vi "Tusk.ValidateName.vi"(8 "error in (no error)":errorcluster, 10 "Name":string, 11 "Tusk in":refnum<class "Tusk.lvclass">) -> (0 "error out":errorcluster, 3 "Tusk out":refnum<class "Tusk.lvclass">)   [LabVIEW 2018, in "Application.lvlib" / "Tusk.lvclass"]
uses:
  Tusk.lvclass
  Exceptions Class/Exceptions.lvclass
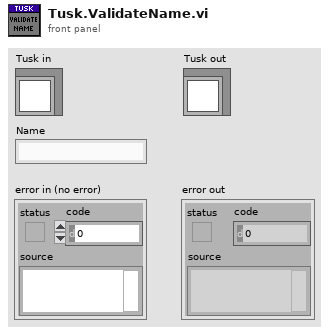
[diagram p1: front panel]
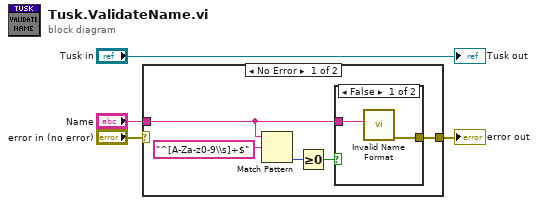
[diagram p0: block diagram]
diagram:
  n1 = case shown="No Error" "error in (no error)" {
    selector: "error in (no error)" -> [_ w12]
    tunnel: [w5 w12] -> w3
    tunnel: "Name" -> [w6 _]
    frame No Error {
      n2 = Match Pattern(string=w6, regular expression="^[A-Za-z0-9\\s]+$") -> (offset past match=w9:i32)  [unwired: 1 in, 3 out]
      n3 = Greater Or Equal To 0?(x=w9) -> (x >= 0?=w7:bool)
      n4 = case shown="False" w7 {
        tunnel: w6 -> [w11 _]
        tunnel: [w10 _] -> w5
        frame False {
          n5 = call "Invalid Name Format.vi"("Name"=w11) -> ("error out"=w10:errorcluster)  [unwired: 10 in]
        }
        frame True {
        }
      }
    }
    frame Error {
    }
  }
  "error out" <- w3
  "Tusk out" <- "Tusk in"
